vi "File Handler object.vi"(8 "error in (no error)":errorcluster, 9 "Image":T1, 10 "Frames":u16, 11 "Start":bool) -> (0 "error out":errorcluster)   [LabVIEW 2015]
uses:
  <vilib>/vision/Image Controls.llb/IMAQ Image.ctl
  Stream/LP Globals.vi
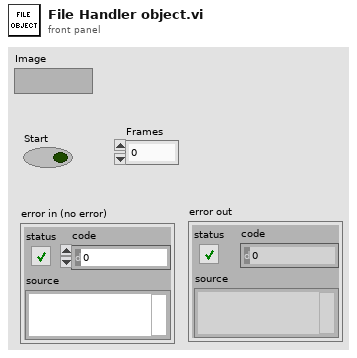
[diagram p1: front panel]
types:
  T1 = typedef "IMAQ Image.ctl" = refnum<image>
  T2 = enum16{"Idle", "OpenFile", "WriteFrame", "CloseFile"}
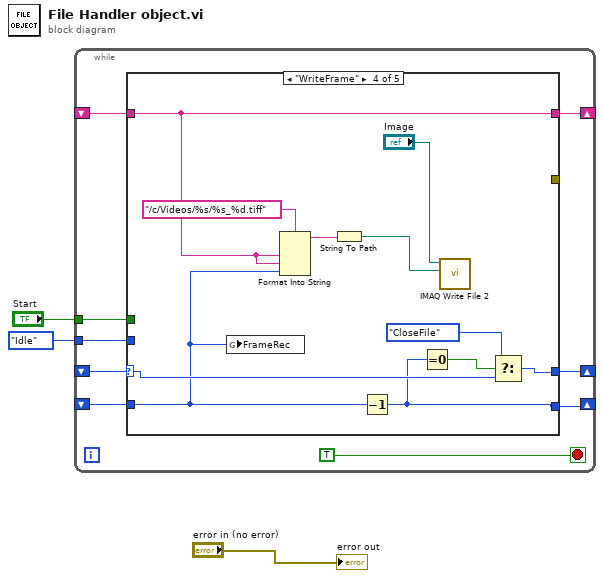
[diagram p0: block diagram]
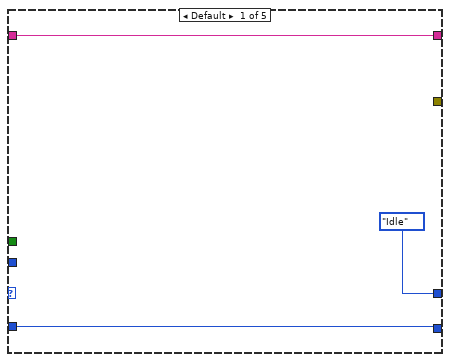
[diagram p2: hidden frame]
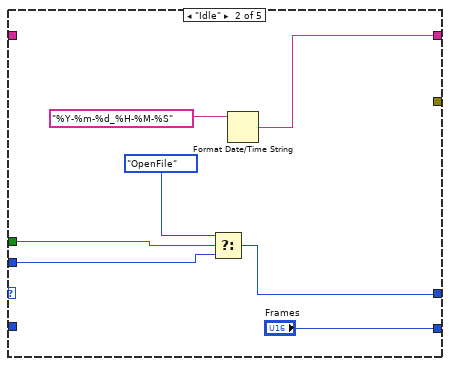
[diagram p3: hidden frame]
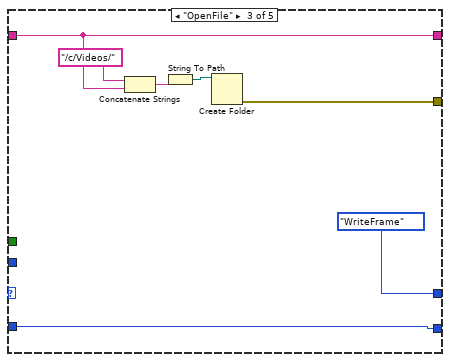
[diagram p4: hidden frame]
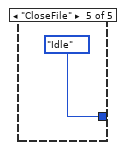
[diagram p5: hidden frame]
diagram:
  n1 = while {
    shift-right: [w10] -> _
    shift-left: _ -> [w12]
    tunnel: T2."Idle" ("AVI_CMD") -> [w9]
    tunnel: "Start" -> [w8]
    shift-right: [w7] -> _
    shift-left: _ -> [w6]
    shift-right: [w5] -> _
    shift-left: _ -> [w4]
    stop <- TRUE stop-if-true
    n2 = case shown="\"WriteFrame\"" w12 {
      selector: w12 -> [_ _ _ w38 _]
      tunnel: [T2."Idle" ("AVI_CMD") w21 T2."WriteFrame" ("AVI_CMD") w34 T2."Idle" ("AVI_CMD")] -> w10
      tunnel: w9 -> [_ w22 _ _ _]
      tunnel: w8 -> [_ w20 _ _ _]
      tunnel: [w14 w16 w24 w32 _] -> w7
      tunnel: w6 -> [w14 _ w24 w32 _]
      tunnel: [w13 "Frames" w27 w37 _] -> w5
      tunnel: w4 -> [w13 _ w27 w30 _]
      tunnel: [_ _ w26 _ _] -> _
      frame Default {
      }
      frame "Idle" {
        n3 = Select(t=T2."OpenFile", s=w20, f=w22) -> (s? t:f=w21:T2)
        n4 = Format Date/Time String(time format string (%c)="%Y-%m-%d_%H-%M-%S") -> (date/time string=w16:string)  [unwired: 2 in]
      }
      frame "OpenFile" {
        n5 = Concatenate Strings("/c/Videos/" ("string"), w24) -> (w23:string)
        n6 = String To Path(string=w23) -> (path=w28:path)
        n7 = Create Folder(path (use dialog)=w28) -> (error out=w26:errorcluster)  [unwired: 2 in, 2 out]
      }
      frame "WriteFrame" {
        n8 = global write "LP Globals.vi" "FrameRec"(w30) -> ()
        n9 = Format Into String(format string="/c/Videos/%s/%s_%d.tiff", w32, w32, w30) -> (resulting string=w31:string)  [unwired: 2 in, 1 out]
        n10 = String To Path(string=w31) -> (path=w40:path)
        n11 = Decrement(x=w30) -> (x-1=w37:u16)
        n12 = Equal To 0?(x=w37) -> (x = 0?=w36:bool)
        n13 = call-poly "IMAQ Write File 2"("File Path"=w40, "Image"="Image") -> ()  [unwired: 8 in, 2 out]
        n14 = Select(t=T2."CloseFile", s=w36, f=w38) -> (s? t:f=w34:T2)
      }
      frame "CloseFile" {
      }
    }
  }
  "error out" <- "error in (no error)"
